vi "myRIO_BRig_RT_dataCurrent_Tcycle_reward.vi"() -> (2 "output_Tcycle_reward":i32)   [LabVIEW 2014]
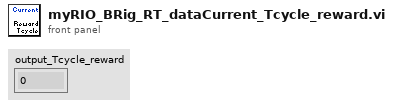
[diagram p1: front panel]
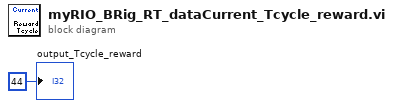
[diagram p0: block diagram]
diagram:
  "output_Tcycle_reward" <- 44 ("output_iBlock")
